vi "GetAvailableResolutions.vi"(8 "error in (no error)":errorcluster, 11 "dResolutions":dbl) -> (0 "error out":errorcluster, 2 "function return":i16, 3 "dResolutions out":dbl)   [LabVIEW 2013, in "HS3OverallRoutines.lvlib"]
doc: "The Handyscope HS3 and Handyscope HS4 support different,\nuser selectable input resolutions. This routine retrieves the available input resolutions from the hardware and stores them in an array. dResolutions is a 20 elements large array. The caller must ensure that there is enough space in the array to contain the data. Therefore the size of the array in bytes must be at least 20 * sizeof(double). At return, all elements containing a non-zero value, contain an input resolution in number of bits.\n\ninput: -\noutput: dResolutions the array of input sensitivities\nReturn value E_NO_ERRORS | E_NO_HARDWARE\n\nFunction prototype: word GetAvailableResolutions( double *dResolutions )\n\nshort int GetAvailableResolutions ( double *dResolutions );"
uses:
  HS3OverallRoutines.lvlib
  hs3.dll
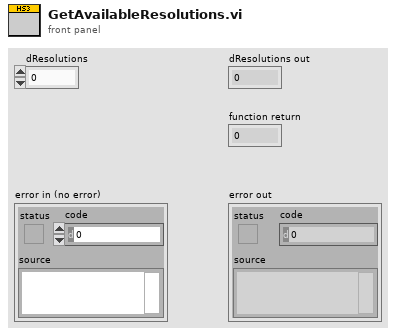
[diagram p1: front panel]
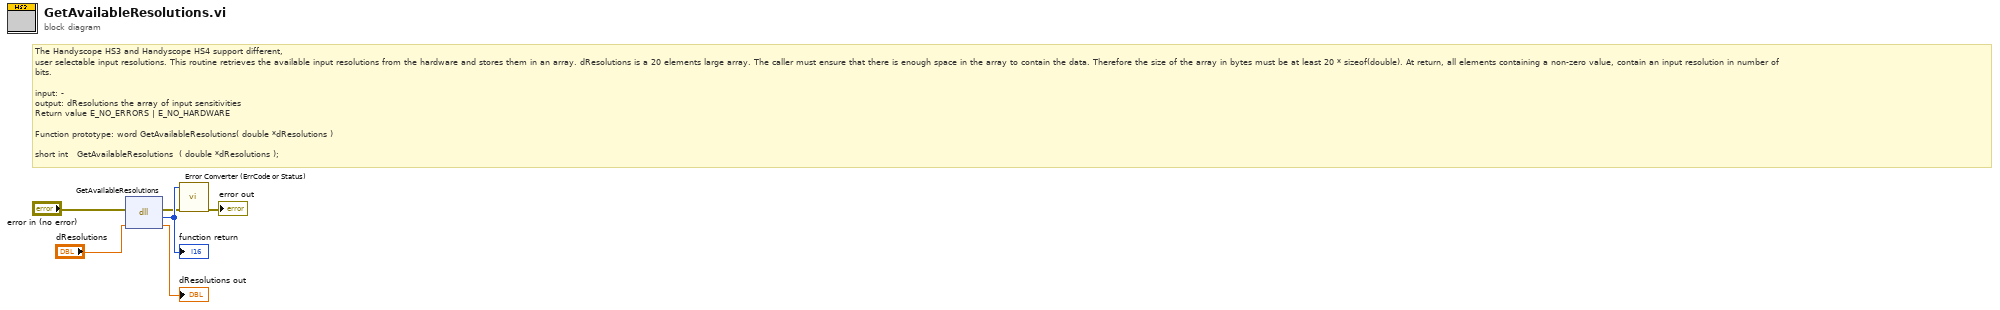
[diagram p0: block diagram]
diagram:
  # "The Handyscope HS3 and Handyscope HS4 support different,\nuser selectable input resolutions. This routine retrieves the available input resolutions from the hardware and stores them in an array. dResolutions is a 20 elements large array. The caller must ensure that there is enough space in the array to contain the data. Therefore the size of the array in bytes must be at least 20 * sizeof(double). At return, all elements containing a non-zero value, contain an input resolution in number of bits.\n\ninput: -\noutput: dResolutions the array of input sensitivities\nReturn value E_NO_ERRORS | E_NO_HARDWARE\n\nFunction prototype: word GetAvailableResolutions( double *dResolutions )\n\nshort int \t\tGetAvailableResolutions\t\t( double *dResolutions );"
  n1 = dll-call lib="C:/Documents and Settings/admin/Pulpit/HS3 LabViewLib/HS3_WRAPPER/OverallRoutines/hs3.*" fn="GetAvailableResolutions"(error in="error in (no error)", "dResolutions"="dResolutions") -> (error out=w2:errorcluster, w6:i16, "dResolutions"=→"dResolutions out":dbl)  [unwired: 2 in, 1 out]
  "function return" <- w6
  n2 = call "Error Converter (ErrCode or Status).vi"("error in (no error)"=w2, "error code"=w6) -> ("error out"=→"error out":errorcluster)  [unwired: 9 in]
